vi "Set 2D Array Double.vi"(5 "use temporary file? (F)":bool, 8 "error in":errorcluster, 9 "value":dbl[][](array[numeric]), 10 "variable name":string, 11 "GOLPI ref. in":T1={"pipe handle"={"lv_proc.dll file path"=path "", "process instance handle"=[], "debug mode"=FALSE, "debug data"=[]}, "fast read timeout [ms]"=500, "fast read settle time [ms]"=10, "fast read to multiple [ms]"=1, "max elements per input line"=100, "slow read timeout [ms]"=5000, "stdin double format specifier"="%_16e", "max elements per stdout output column"=100, "console mode bitstream"=FALSE, "bitstream first read timeout [ms]"=1000, "bitstream read timeout [ms]"=50, "struct transfer possible"=FALSE, "matlab mode"=FALSE}) -> (0 "error out":errorcluster, 3 "GOLPI ref. out":T1={"pipe handle"={"lv_proc.dll file path"=path "", "process instance handle"=[], "debug mode"=FALSE, "debug data"=[]}, "fast read timeout [ms]"=500, "fast read settle time [ms]"=10, "fast read to multiple [ms]"=1, "max elements per input line"=100, "slow read timeout [ms]"=5000, "stdin double format specifier"="%_16e", "max elements per stdout output column"=100, "console mode bitstream"=FALSE, "bitstream first read timeout [ms]"=1000, "bitstream read timeout [ms]"=50, "struct transfer possible"=FALSE, "matlab mode"=FALSE})   [LabVIEW 2020, in "GOLPI library.lvlib"]
doc: "Part of polymorph Set Variable.vi"
uses:
  GOLPI library.lvlib
  GOLPI reference Type Def.ctl
  Pipe Handle.ctl
  LV Process library.lvlib
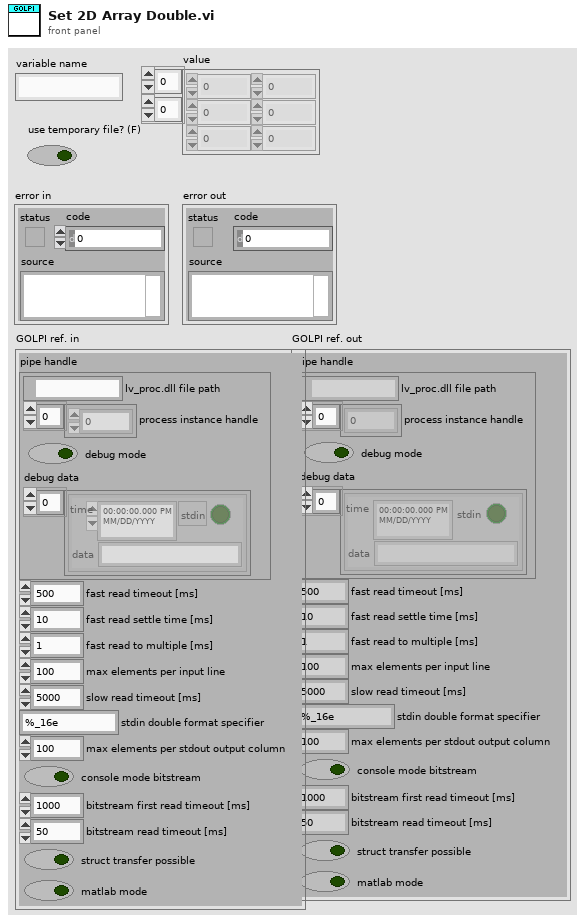
[diagram p1: front panel]
types:
  T1 = typedef "GOLPI library.lvlib/GOLPI reference Type Def.ctl" = cluster{"pipe handle":T2, "fast read timeout [ms]":u32, "fast read settle time [ms]":u32, "fast read to multiple [ms]":u32, "max elements per input line":u32, "slow read timeout [ms]":u32, "stdin double format specifier":string, "max elements per stdout output column":u32, "console mode bitstream":bool, "bitstream first read timeout [ms]":u32, "bitstream read timeout [ms]":u32, "struct transfer possible":bool, "matlab mode":bool}
  T2 = typedef "LV Process library.lvlib/Pipe Handle.ctl" = cluster{"lv_proc.dll file path":path, "process instance handle":u32[], "debug mode":bool, "debug data":cluster{"time":timestamp, "stdin":bool, "data":string}[]}
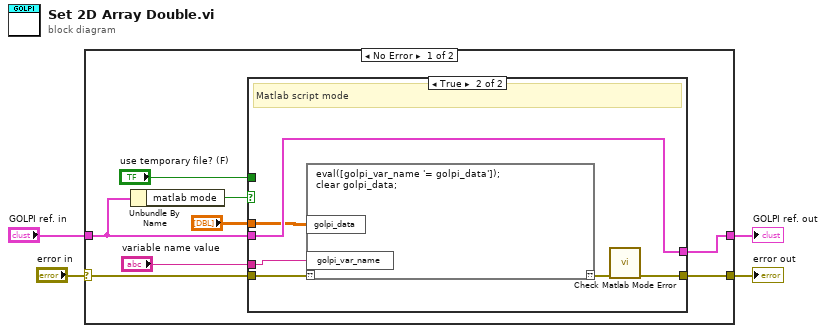
[diagram p0: block diagram]
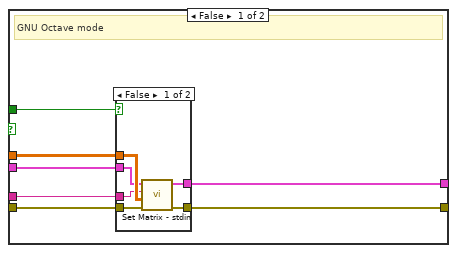
[diagram p2: hidden frame]
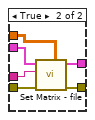
[diagram p3: hidden frame]
diagram:
  n1 = case shown="No Error" "error in" {
    selector: "error in" -> [w10 w39]
    tunnel: [w9 w39] -> w4
    tunnel: "GOLPI ref. in" -> [w6 w38]
    tunnel: [w8 w38] -> w1
    frame No Error {
      n2 = Unbundle By Name(w6) -> ("matlab mode"=w5:bool)
      n3 = case shown="True" w5 {
        tunnel: "value" -> [w19 w35]
        tunnel: "variable name" -> [w18 w34]
        tunnel: w10 -> [w17 w37]
        tunnel: [w16 w32] -> w9
        tunnel: w6 -> [w15 w36]
        tunnel: [w14 w36] -> w8
        tunnel: "use temporary file? (F)" -> [w13 _]
        frame False {
          # "GNU Octave mode"
          n4 = case shown="False" w13 {
            tunnel: w19 -> [w25 w26]
            tunnel: w18 -> [w24 w27]
            tunnel: w17 -> [w23 w31]
            tunnel: [w22 w30] -> w16
            tunnel: w15 -> [w21 w28]
            tunnel: [w20 w29] -> w14
            frame False {
              n5 = call "Set Matrix - stdin.vi"("error in"=w23, "value"=w25, "variable name"=w24, "GOLPI ref. in"=w21) -> ("error out"=w22:errorcluster, "GOLPI ref. out"=w20:T1)  [unwired: 6 in]
            }
            frame True {
              n6 = call "Set Matrix - file.vi"("double array"=w26, "error in (no error)"=w31, "variable name"=w27, "GOLPI ref. in"=w28) -> ("error out"=w30:errorcluster, "GOLPI ref. out"=w29:T1)  [unwired: 6 in]
            }
          }
        }
        frame True {
          # "Matlab script mode"
          n7 = script code="eval([golpi_var_name '= golpi_data']);\nclear golpi_data;"("??"=w37, "golpi_var_name"=w34, "golpi_data"=w35) -> ("??"=w33:errorcluster)
          n8 = call "Check Matlab Mode Error.vi"("error in"=w33) -> ("error out"=w32:errorcluster)  [unwired: 10 in]
        }
      }
    }
    frame Error {
    }
  }
  "error out" <- w4
  "GOLPI ref. out" <- w1
